vi "Should Stop.vi"(0 "error in 1":errorcluster, 1 "error in 2":errorcluster, 2 "Stop Button":bool, 3 "Look at Stop Button":bool, 4 "Initialize":bool) -> (5 "error out":errorcluster, 6 "Stop":bool)   [LabVIEW 2020]
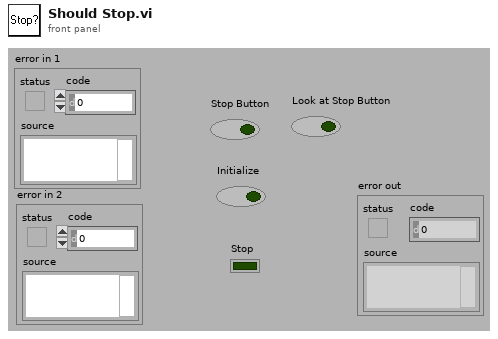
[diagram p1: front panel]
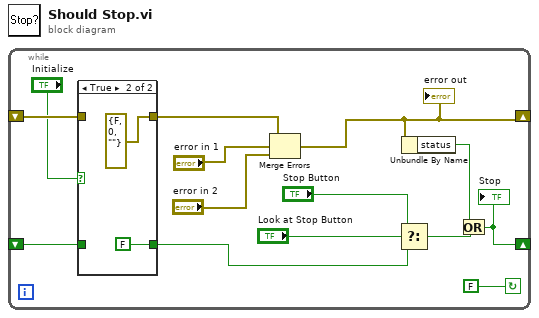
[diagram p0: block diagram]
diagram:
  n1 = while {
    shift-right: [w7] -> _
    shift-left: _ -> [w4]
    shift-right: [w6] -> _
    shift-left: _ -> [w5]
    stop <- FALSE continue-if-true
    n2 = case shown="True" "Initialize" {
      tunnel: w5 -> [w16 _]
      tunnel: w4 -> [w15 _]
      tunnel: [w15 FALSE] -> w3
      tunnel: [w16 errorcluster {"status"=FALSE, "code"=0, "source"=""} ("error out")] -> w2
      frame False {
      }
      frame True {
      }
    }
    n3 = Merge Errors(w2, "error in 1", "error in 2") -> (w6:errorcluster)
    "error out" <- w6
    n4 = Select(t="Stop Button", s="Look at Stop Button", f=w3) -> (s? t:f=w8:bool)
    n5 = Unbundle By Name(w6) -> ("status"=w9:bool)
    n6 = Or(x=w9, y=w8) -> (x .or. y?=w7:bool)
    "Stop" <- w7
  }
